vi "test-wrl read.vi"() -> ()   [LabVIEW 2013]
uses:
  <vilib>/Utility/miscctls.llb/LVBoundsTypeDef.ctl
  <vilib>/picture/3D Picture Control/NI_3D Picture Control.lvlib
panel:
  in  "Angle":sgl caption="角"
  in  "Axis":cluster{"X":sgl, "Y":sgl, "Z":sgl} caption="轴"
  out "内容边界":T1
  in  "停止按钮":bool
  out "三维图片":refnum<vi>(3d-picture)
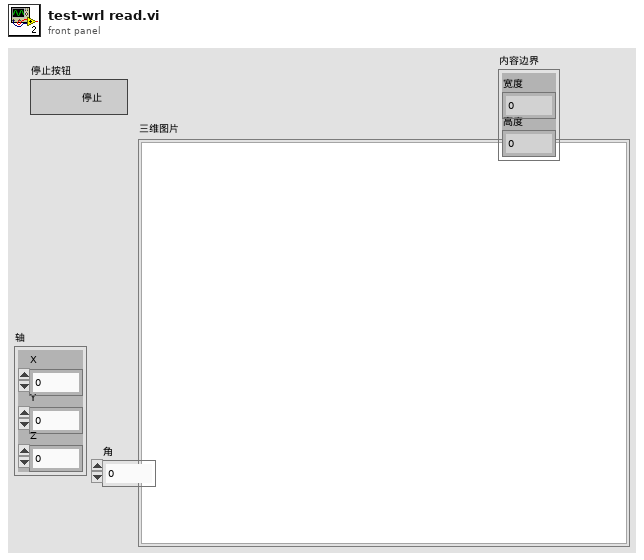
[diagram p1: front panel]
types:
  T1 = typedef "LVBoundsTypeDef.ctl" = cluster{"Width":u32, "Height":u32}
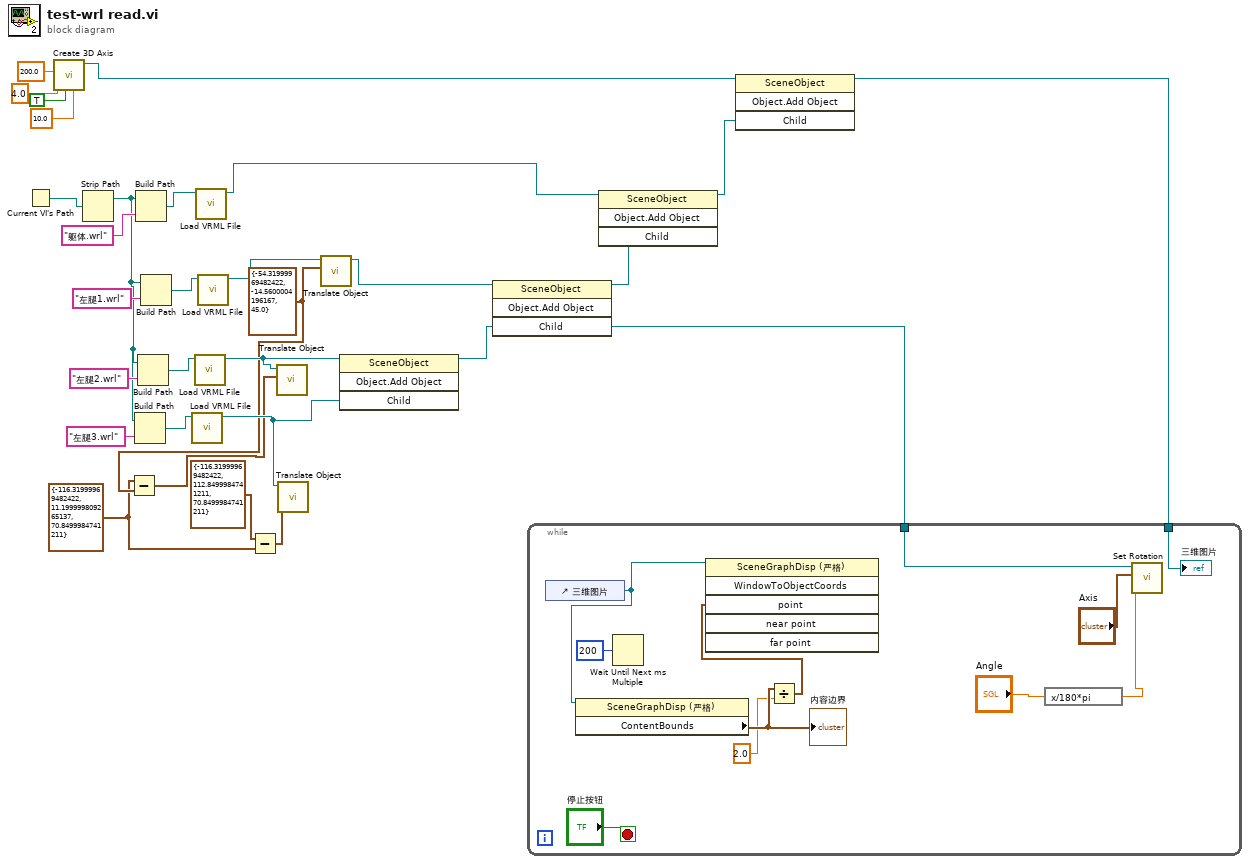
[diagram p0: block diagram]
diagram:
  w7 = cluster{"X":sgl, "Y":sgl, "Z":sgl} {"X"=-54.32, "Y"=-14.56, "Z"=45.0} ("Translation")
  w4 = cluster{"X":sgl, "Y":sgl, "Z":sgl} {"X"=-116.32, "Y"=11.2, "Z"=70.85} ("Translation")
  n1 = Current VI's Path() -> (path=w30:path)
  n2 = call <vilib>:"Create 3D Axis.vi"("Character Size"=sgl 10.0, "Axis label?"=TRUE, "Radius"=sgl 4.0, "Length"=sgl 200.0) -> ("New Object Refnum"=w23:refnum<vi>)  [unwired: 6 in, 1 out]
  n3 = Strip Path(path=w30) -> (stripped path=w14:path)  [unwired: 1 out]
  n4 = Subtract(x=w4, y=w7) -> (x-y=w6:cluster{"X":sgl, "Y":sgl, "Z":sgl})
  n5 = Build Path(base path=w14, name or relative path="左腿3.wrl" ("名称或相对路径")) -> (appended path=w18:path)
  n6 = Build Path(base path=w14, name or relative path="躯体.wrl" ("名称或相对路径")) -> (appended path=w29:path)
  n7 = Build Path(base path=w14, name or relative path="左腿2.wrl" ("名称或相对路径")) -> (appended path=w25:path)
  n8 = Build Path(base path=w14, name or relative path="左腿1.wrl" ("名称或相对路径")) -> (appended path=w26:path)
  n9 = call <vilib>:"Load VRML File.vi"("Path"=w18) -> ("Scene:Read Scene File"=w8:refnum<vi>)  [unwired: 9 in, 1 out]
  n10 = call <vilib>:"Load VRML File.vi"("Path"=w25) -> ("Scene:Read Scene File"=w9:refnum<vi>)  [unwired: 9 in, 1 out]
  n11 = call <vilib>:"Load VRML File.vi"("Path"=w29) -> ("Scene:Read Scene File"=w17:refnum<vi>)  [unwired: 9 in, 1 out]
  n12 = call <vilib>:"Load VRML File.vi"("Path"=w26) -> ("Scene:Read Scene File"=w12:refnum<vi>)  [unwired: 9 in, 1 out]
  n13 = Subtract(x=cluster{"X":sgl, "Y":sgl, "Z":sgl} {"X"=-116.32, "Y"=112.85, "Z"=70.85} ("Translation"), y=w4) -> (x-y=w3:cluster{"X":sgl, "Y":sgl, "Z":sgl})
  n14 = call <vilib>:"Translate Object.vi"("Translation"=w6, "Scene.Object In"=w9) -> ()  [unwired: 8 in, 2 out]
  n15 = call <vilib>:"Translate Object.vi"("Translation"=w3, "Scene.Object In"=w8) -> ()  [unwired: 8 in, 2 out]
  n16 = call <vilib>:"Translate Object.vi"("Translation"=w7, "Scene.Object In"=w12) -> ("Scene.Object Out"=w11:refnum<vi>)  [unwired: 8 in, 1 out]
  n17 = invoke class="SceneObject" method="Object.Add Object"(reference=w9, "Child"=w8) -> (reference out=w10:refnum<vi>)  [unwired: 2 in, 3 out]
  n18 = invoke class="SceneObject" method="Object.Add Object"(reference=w11, "Child"=w10) -> (reference out=w16:refnum<vi>, "Child"=w1:refnum<vi>)  [unwired: 2 in, 2 out]
  n19 = invoke class="SceneObject" method="Object.Add Object"(reference=w17, "Child"=w16) -> (reference out=w15:refnum<vi>)  [unwired: 2 in, 3 out]
  n20 = invoke class="SceneObject" method="Object.Add Object"(reference=w23, "Child"=w15) -> (reference out=w2:refnum<vi>)  [unwired: 2 in, 3 out]
  n21 = while {
    tunnel: w1 -> [w32]
    tunnel: w2 -> [w31]
    stop <- "停止按钮" stop-if-true
    n22 = control-ref of="三维图片"() -> (w39:refnum<vi>)
    n23 = property class="SceneGraphDisp (严格)"(reference=w39) -> ("ContentBounds"=w38:T1)  [unwired: 1 in, 2 out]
    "内容边界" <- w38
    n24 = Wait Until Next ms Multiple(millisecond multiple=u32 200 ("毫秒倍数")) -> ()  [unwired: 1 out]
    n25 = Divide(x=w38, y=2.0) -> (x/y=w36:cluster{"Width":dbl, "Height":dbl})
    n26 = invoke class="SceneGraphDisp (严格)" method="WindowToObjectCoords"(reference=w39, "point"=w36) -> ()  [unwired: 4 in, 6 out]
    n27 = expression code="x/180*pi"("Angle") -> (w33:sgl)
    n28 = call <vilib>:"Set Rotation.vi"("Angle"=w33, "Axis"="Axis", "Scene Object"=w32) -> ()  [unwired: 7 in, 2 out]
    "三维图片" <- w31
  }
